vi "Digital Read.vi"() -> ()   [LabVIEW 2009]
uses:
  <vilib>/DAQmx/create/channels.llb/DAQmx Create Channel (DI-Digital Input).vi
  <vilib>/DAQmx/read.llb/DAQmx Read (Digital Bool 1Line 1Point).vi
panel:
  in  "lines":tag="Dev1/port0/line7"
  out "data":bool
  in  "stop":bool
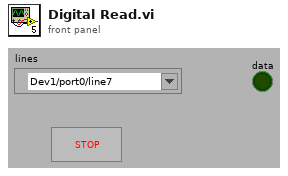
[diagram p1: front panel]
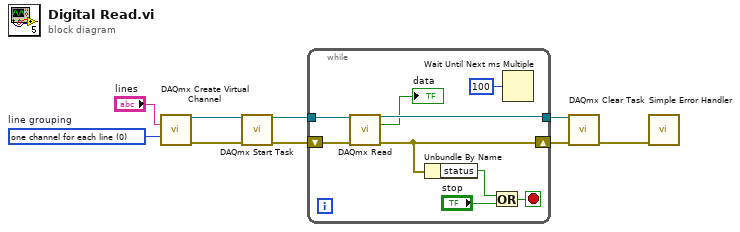
[diagram p0: block diagram]
diagram:
  w2 = 0 items=["one channel for each line", "one channel for all lines"]  # line grouping
  n1 = call-poly <vilib>:"DAQmx Create Virtual Channel.vi"("lines"="lines", "line grouping"=w2) -> ("task out"=w9:refnum<k21>, "error out"=w6:errorcluster)  [unwired: 12 in]
  n2 = call <vilib>:"DAQmx Start Task.vi"("task/channels in"=w9, "error in"=w6) -> ("task out"=w8:refnum<k21>, "error out"=w5:errorcluster)  [unwired: 12 in]
  n3 = while {
    tunnel: w8 -> [w18]
    tunnel: [w17] -> w7
    shift-right: [w15] -> w4
    shift-left: w5 -> [w16]
    stop <- w12 stop-if-true
    n4 = call-poly <vilib>:"DAQmx Read.vi"("task/channels in"=w18, "error in"=w16) -> ("task out"=w17:refnum<k21>, "data"=→"data":bool, "error out"=w15:errorcluster)  [unwired: 11 in]
    n5 = Unbundle By Name "Unbundle By Name"(w15) -> ("status"=w14:bool)
    n6 = Or(x=w14, y="stop") -> (x .or. y?=w12:bool)
    n7 = Wait Until Next ms Multiple(millisecond multiple=u32 100) -> ()  [unwired: 1 out]
  }
  n8 = call <vilib>:"DAQmx Clear Task.vi"("task in"=w7, "error in"=w4) -> ("error out"=w3:errorcluster)  [unwired: 13 in]
  n9 = call <vilib>:"Simple Error Handler.vi"("error in (no error)"=w3) -> ()  [unwired: 4 in, 5 out]
